vi "task 3.vi"() -> ()   [LabVIEW 2017]
uses:
  <vilib>/DAQmx/write.llb/DAQmx Write (Analog DBL 1Chan 1Samp).vi
  <vilib>/DAQmx/create/channels.llb/DAQmx Create Channel (AO-Voltage-Basic).vi
  <vilib>/DAQmx/create/channels.llb/DAQmx Create Channel (DI-Digital Input).vi
  <vilib>/DAQmx/read.llb/DAQmx Read (Digital Bool 1Line 1Point).vi
  <vilib>/DAQmx/read.llb/DAQmx Read (Counter DBL 1Chan 1Samp).vi
  <vilib>/DAQmx/create/channels.llb/DAQmx Create Channel (CI-Count Edges).vi
  <vilib>/Simulation/Implementation/XNodeFramework/SimXNode/SimX.xnode
  <vilib>/Simulation/Model Libraries/PID/SIM PID.vi
  <vilib>/Simulation/Model Libraries/PID/SIM PID (Parallel).vi
  <vilib>/Simulation/Implementation/Shared/SIMSCR Execution Mode.ctl
  <vilib>/Simulation/Scripting/Companion Diagram/SimConfigNode/_simSolvers.ctl
  <vilib>/Simulation/Scripting/Companion Diagram/SimConfigNode/SimParams.ctl
  <vilib>/Simulation/Scripting/Companion Diagram/SimConfigNode/SimDog.xnode
  <vilib>/Simulation/Model Libraries/PID/SIM PID (Academic).vi
  <vilib>/Simulation/Implementation/Shared/SIM Bundle Sim Info.vi
  <vilib>/Simulation/Implementation/Shared/SIM Unbundle Sim Info.vi
  <vilib>/Simulation/Implementation/Shared/NILVSim_FinalizeModel.vi
  <vilib>/Simulation/Implementation/Shared/NILVSim_GetModelError.vi
  <vilib>/Simulation/Implementation/Shared/NILVSim_Initialize.vi
  <vilib>/Simulation/Utility/Implementation/NILVSim Get Time and IsAcceptedStep.vi
  <vilib>/Simulation/Implementation/Shared/NILVSim_Manager.vi
  <vilib>/Simulation/Implementation/Shared/NI_SIM_Implementation.lvlib
  <vilib>/Simulation/Implementation/Shared/NILVSIM_BeginStep.vi
  <vilib>/Simulation/Param Hierarchy/Typedefs/SIMPH Param Control Actions.ctl
  <vilib>/Simulation/Implementation/Shared/NILVSim_ParamChanged.vi
  <vilib>/Utility/error.llb/Clear Errors.vi
  <vilib>/Simulation/Implementation/Shared/SIMSH Read Queue.vi
panel:
  in  "rectrangle":bool
  in  "Circle":bool
  in  "Right-Down":bool
  in  "Left-Up":bool
  in  "Left-Down":bool
  in  "Right-Up":bool
  in  "right":bool
  in  "left":bool
  in  "motor 2":dbl(slide)=1.5 scale=-10.0..10.0
  in  "down":bool
  in  "up":bool
  in  "Numeric 2":dbl
  in  "Numeric":dbl
  in  "DAQmx Physical Channel 8":tag="Dev9/ao0"
  out "no of pulses 2":dbl format="%.2f"
  in  "DAQmx Physical Channel 7":tag="Dev9/ao0"
  out "no of pulses":dbl format="%.2f"
  out "Right":bool
  out "Bottom":bool
  out "Left":bool
  out "Top":bool
  in  "DAQmx Physical Channel 6":tag
  in  "DAQmx Physical Channel 5":tag
  in  "DAQmx Physical Channel 4":tag
  in  "DAQmx Physical Channel 3":tag
  in  "Motor stop":bool
  in  "DAQmx Physical Channel 2":tag="Dev9/ao0"
  in  "max Voltage":dbl
  in  "Min Voltage":dbl
  in  "DAQmx Physical Channel":tag="Dev9/ao0"
  in  "motor 1":dbl(slide)=1.5 scale=-10.0..10.0
  in  "stop":bool
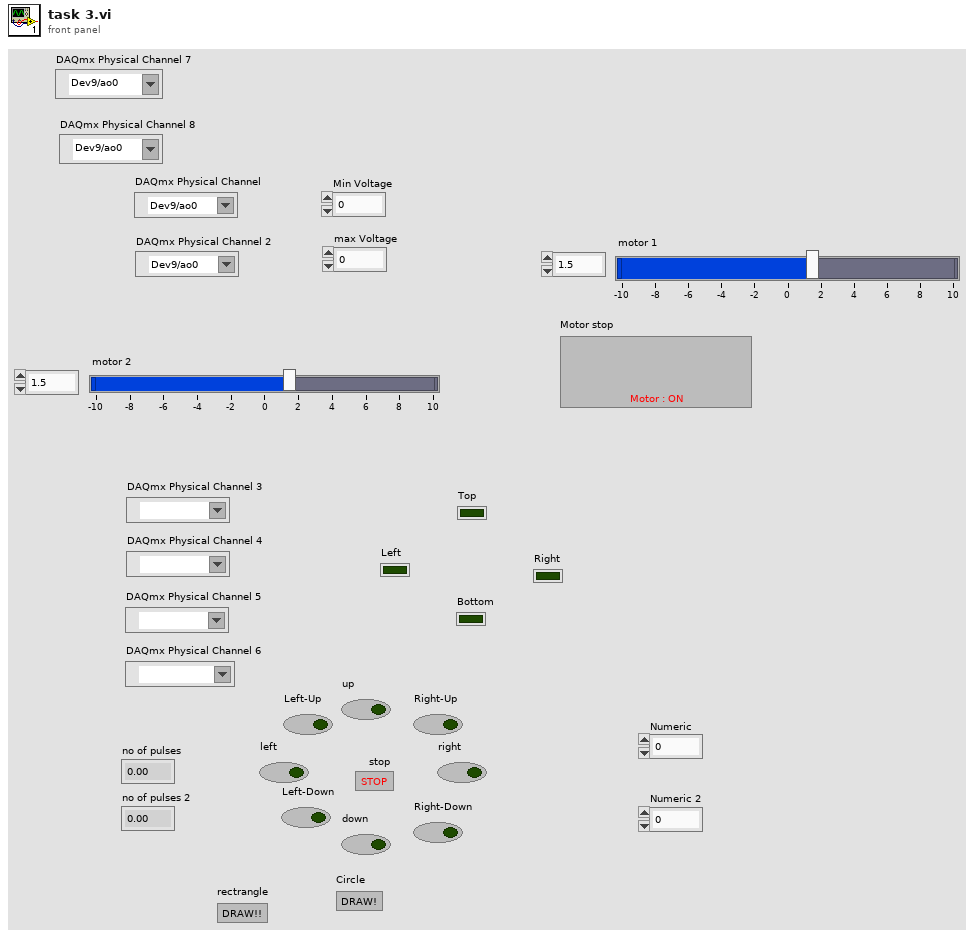
[diagram p1: front panel]
types:
  T1 = enum16{"Simulate to Completion", "Single Time-Step Simulation (Fixed Step Only)"}
  T2 = typedef "SIMSCR Execution Mode.ctl" = enum16{"Simulate to Completion", "Single Time-Step Simulation (Fixed Step Only)"}
  T3 = typedef "SIMPH Param Control Actions.ctl" = enum16{"get params", "set params"}
  T4 = cluster{"SIMSH Sim Time":dbl, "SIM PID Derivative Gain.vi":cluster{"output":dbl}, "SIM PID Derivative Gain.vi - SIMSH":cluster{"SIMSH Sim Time":dbl, "t 3":dbl, "Select 2":cluster{"s? t:f":dbl}, "Equal?":cluster{"x = y?":bool}, "Or":cluster{"x .or. y?":bool}, "Equal To 0?":cluster{"x = 0?":bool}}, "High Frequency [s] (Tf)":dbl, "Gain":cluster{"output":dbl}, "Summation":cluster{"Result":dbl}, "Integral Gain - series.vi":cluster{"output":dbl}, "Integral Gain - series.vi - SIMSH":cluster{"SIMSH Sim Time":dbl, "Select 2":cluster{"s? t:f":dbl}, "integral in gain?":bool, "Integrator":cluster{"output y(t)":dbl}, "Gain 2":cluster{"output":dbl}, "Select":cluster{"s? t:f":dbl}, "Equal To 0?":cluster{"x = 0?":bool}, "Reciprocal":cluster{"1/x":dbl}}}
  T5 = typedef "SimParams.ctl" = cluster{"Initial Time (s)":dbl, "Final Time (s)":dbl, "Step Size (s)":dbl, "ODE Solver":T6, "Minimum Step Size (s)":dbl, "Maximum Step Size (s)":dbl, "Relative Tolerance":dbl, "Absolute Tolerance":dbl, "Software Timing":bool, "Initial Step Size (s)":dbl, "Automatic Fixed Step Size?":bool, "Automatic Discrete Step Size?":bool, "Discrete Step Size (s)":dbl, "Calculate using Time Step":bool, "Solver Wired?":bool, "Prev.Frm.Expected End":u64, "Prev.Frm.Actual End":u64, "Prev.Frm.Finished Late?":bool, "Prev.Iter.Expected End":u64, "Prev.Iter.Actual End":u64, "Prev.Iter.Finished Late?":bool, "Expected Iteration Start":u64, "Actual Iteration Start":u64, "Expected Frame Start":u64, "Actual Frame Start":u64, "Source Name":string, "Name":string, "Period":i64, "Deadline":i64, "Offset":i64, "Start":i64, "Priority":i32, "Timeout":i32, "Processor":i32, "Mode":enum32{"No Change", "Process missed periods, maintain original phase", "Discard missed periods, maintain original phase", "Process missed periods, ignore original phase", "Discard missed periods, ignore original phase"}, "Wakeup reason":enum32{"Normal", "Aborted", "Asynchronous wakeup", "Timing source error", "Timed loop error", "Timeout"}, "Error":errorcluster, "Source Type":string, "Secondary Source Type":string, "Global End Time":u64, "Global Start Time":u64, "Full Solver Reset":bool, "Execution Mode":T2, "Nan/Inf Check":bool, "Custom Solver Library":string, "Solver Is Variable":bool, "custom solver name":string, "Signal Collection Decimation":u32}
  T6 = typedef "_simSolvers.ctl" = enum16{"Runge-Kutta 1 (Euler)", "Runge-Kutta 2", "Runge-Kutta 3", "Runge-Kutta 4", "Runge-Kutta 23 (variable)", "Runge-Kutta 45 (variable)", "BDF (variable)", "Adams-Moulton (variable)", "Rosenbrock (variable)", "Discrete States Only", "SDIRK 4 (variable)", "Radau 5 (variable)", "Radau 9 (variable)", "Radau 13 (variable)", "Radau [Variable Order] (variable)", "Gear's Method (variable)", "Linearizer", "State Query", "Trim Eval", "Custom Solver"}
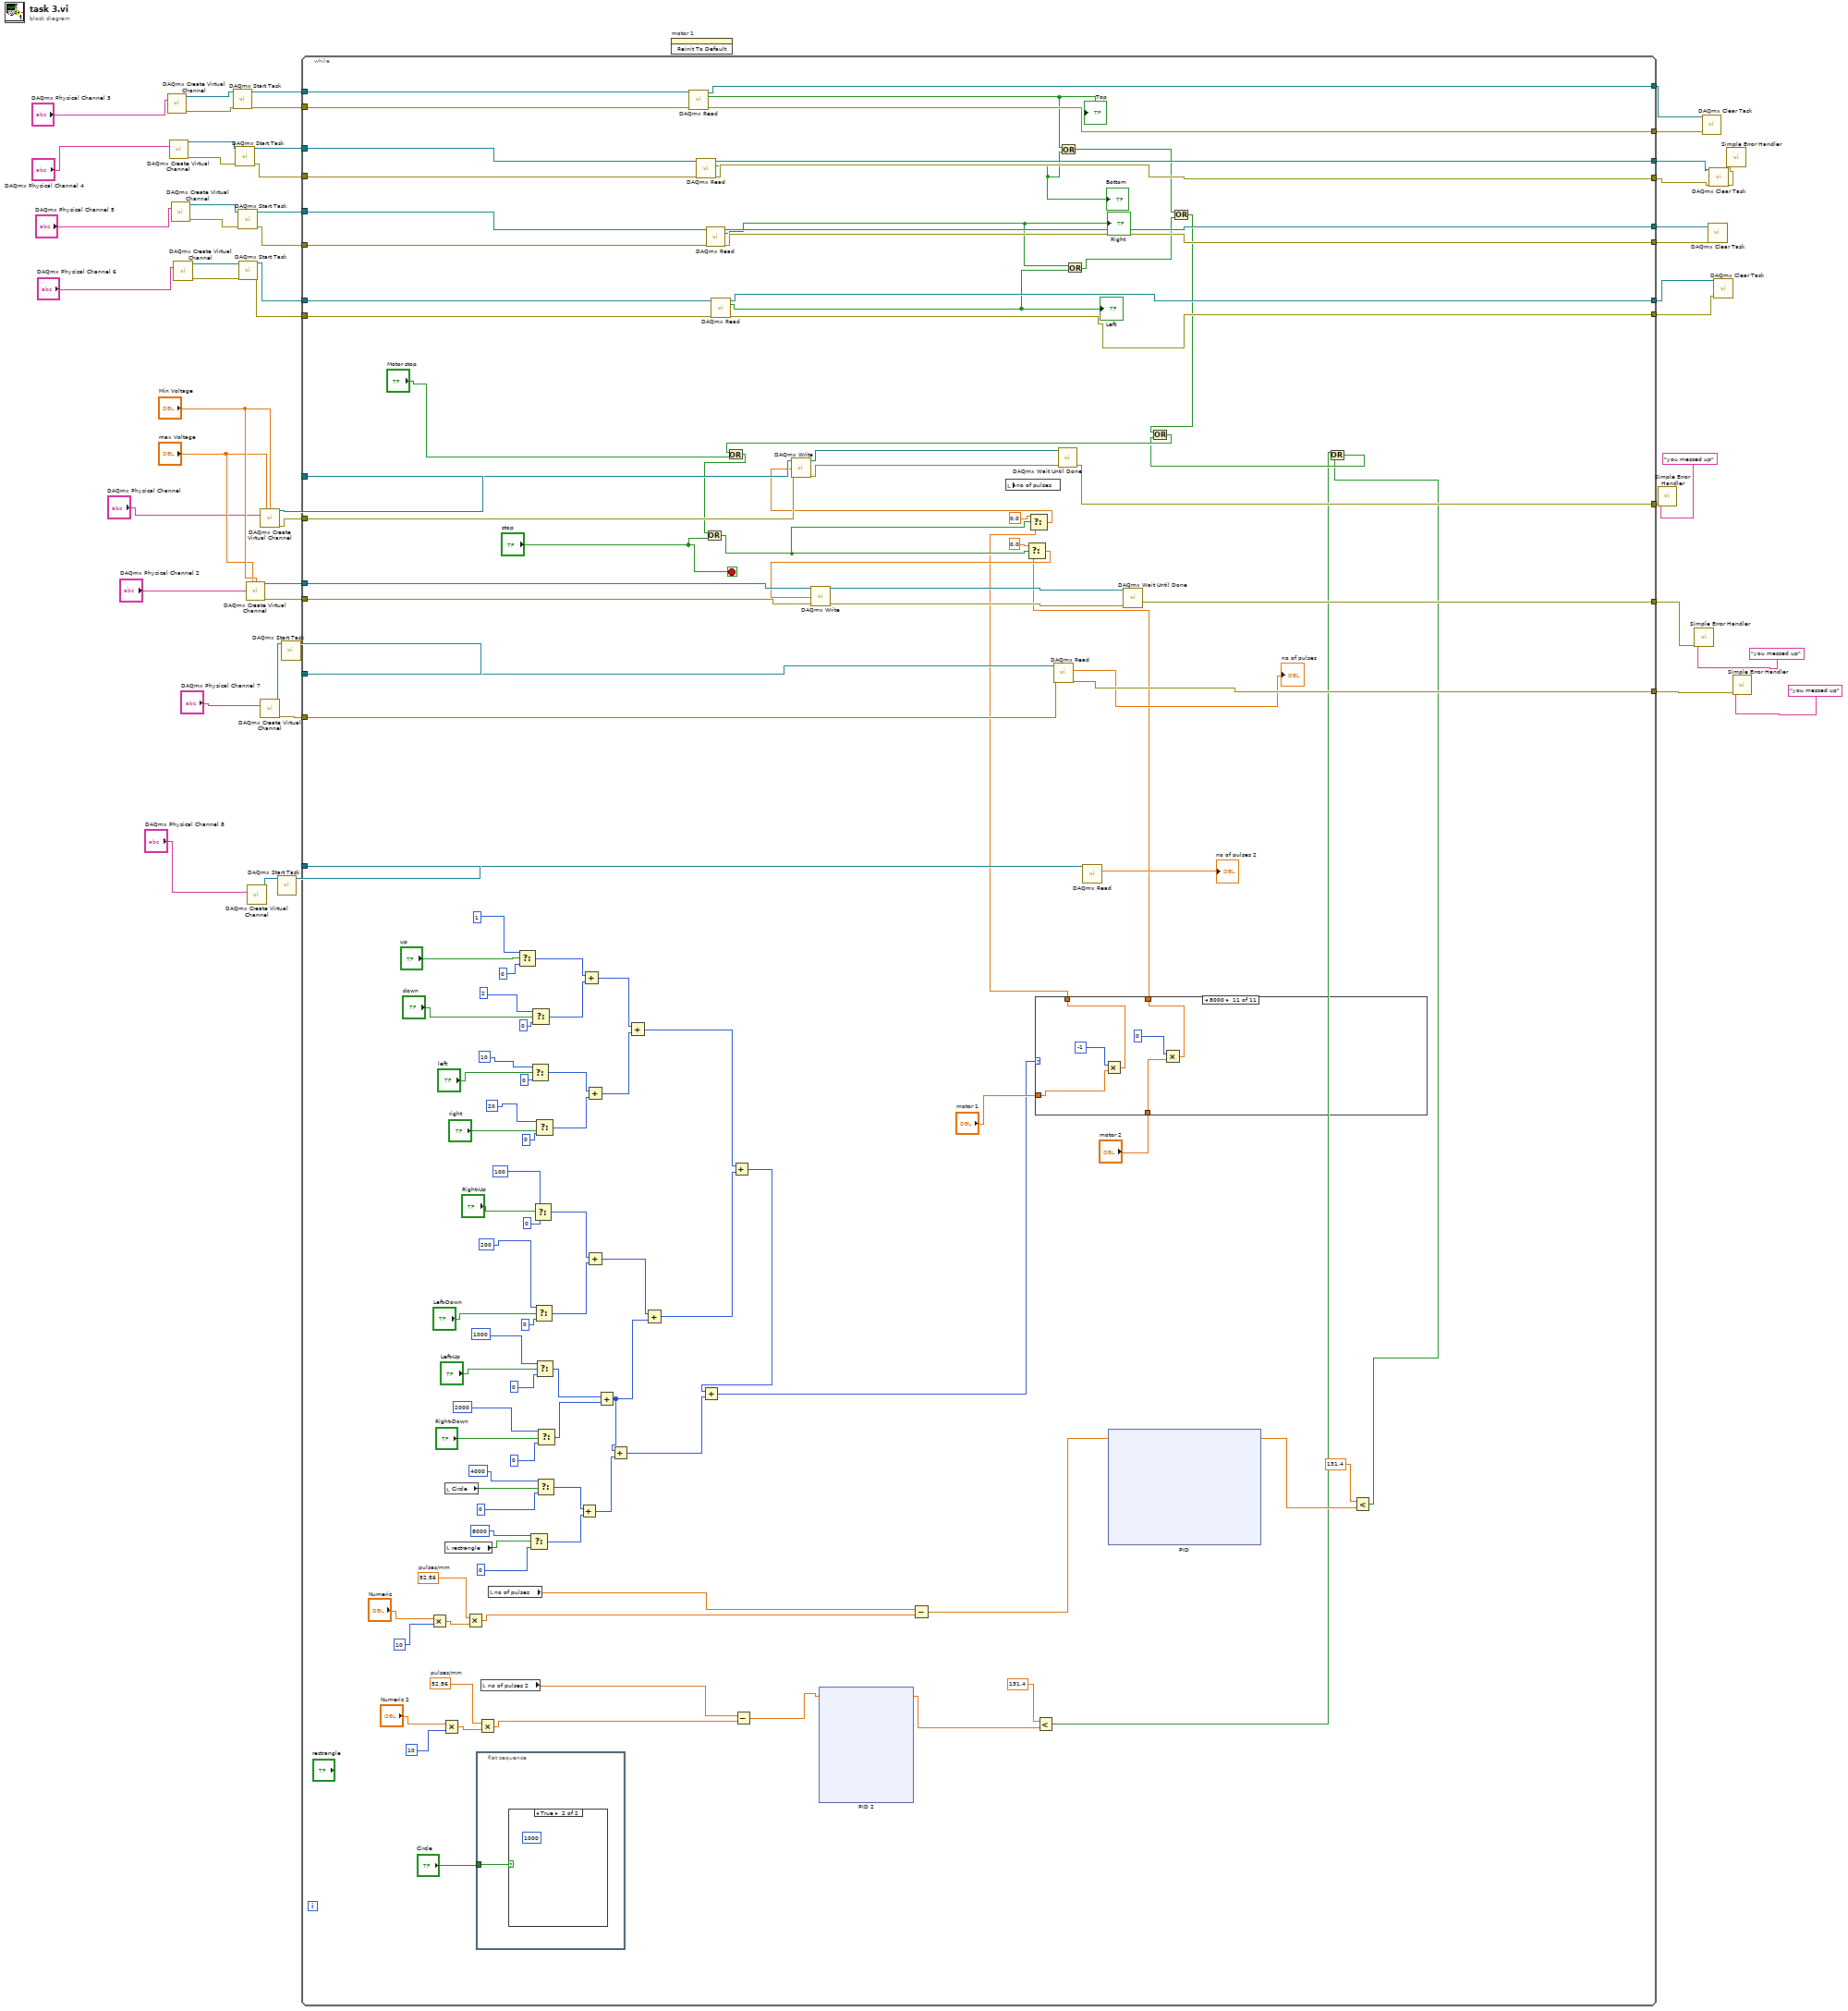
[diagram p0: block diagram]
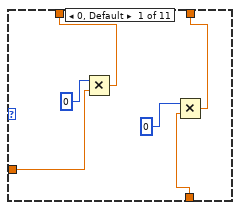
[diagram p3: hidden frame]
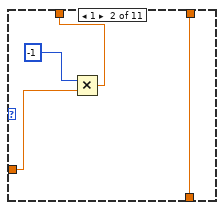
[diagram p4: hidden frame]
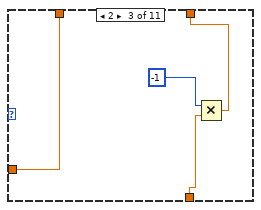
[diagram p5: hidden frame]
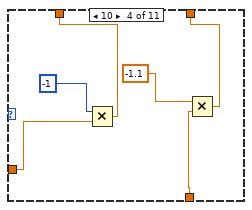
[diagram p6: hidden frame]
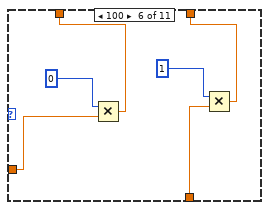
[diagram p8: hidden frame]
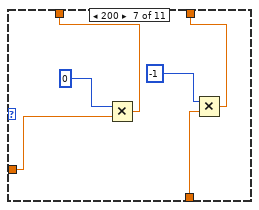
[diagram p9: hidden frame]
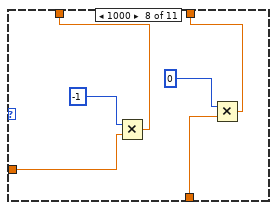
[diagram p10: hidden frame]
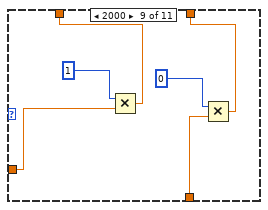
[diagram p11: hidden frame]
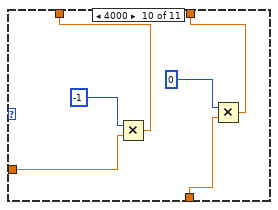
[diagram p12: hidden frame]
diagram:
  n1 = call-poly <vilib>:"DAQmx Create Virtual Channel.vi"("lines"="DAQmx Physical Channel 3") -> ("task out"=w36:refnum<k21>, "error out"=w32:errorcluster)  [unwired: 13 in]
  n2 = call-poly <vilib>:"DAQmx Create Virtual Channel.vi"("lines"="DAQmx Physical Channel 4") -> ("task out"=w35:refnum<k21>, "error out"=w31:errorcluster)  [unwired: 13 in]
  n3 = call-poly <vilib>:"DAQmx Create Virtual Channel.vi"("lines"="DAQmx Physical Channel 5") -> ("task out"=w34:refnum<k21>, "error out"=w30:errorcluster)  [unwired: 13 in]
  n4 = call-poly <vilib>:"DAQmx Create Virtual Channel.vi"("lines"="DAQmx Physical Channel 6") -> ("task out"=w33:refnum<k21>, "error out"=w29:errorcluster)  [unwired: 13 in]
  n5 = call <vilib>:"DAQmx Start Task.vi"("task/channels in"=w36, "error in"=w32) -> ("task out"=w28:refnum<k21>, "error out"=w26:errorcluster)  [unwired: 12 in]
  n6 = call <vilib>:"DAQmx Start Task.vi"("task/channels in"=w35, "error in"=w31) -> ("task out"=w24:refnum<k21>, "error out"=w21:errorcluster)  [unwired: 12 in]
  n7 = call <vilib>:"DAQmx Start Task.vi"("task/channels in"=w34, "error in"=w30) -> ("task out"=w23:refnum<k21>, "error out"=w20:errorcluster)  [unwired: 12 in]
  n8 = call <vilib>:"DAQmx Start Task.vi"("task/channels in"=w33, "error in"=w29) -> ("task out"=w22:refnum<k21>, "error out"=w19:errorcluster)  [unwired: 12 in]
  n9 = call-poly <vilib>:"DAQmx Create Virtual Channel.vi"("maximum value"="max Voltage", "minimum value"="Min Voltage", "physical channels"="DAQmx Physical Channel 2") -> ("task out"=w46:refnum<k21>, "error out"=w42:errorcluster)  [unwired: 11 in]
  n10 = call-poly <vilib>:"DAQmx Create Virtual Channel.vi"("counter"="DAQmx Physical Channel 8") -> ("task out"=w4:refnum<k21>)  [unwired: 13 in, 1 out]
  n11 = call-poly <vilib>:"DAQmx Create Virtual Channel.vi"("maximum value"="max Voltage", "minimum value"="Min Voltage", "physical channels"="DAQmx Physical Channel") -> ("task out"=w49:refnum<k21>, "error out"=w41:errorcluster)  [unwired: 11 in]
  n12 = call-poly <vilib>:"DAQmx Create Virtual Channel.vi"("counter"="DAQmx Physical Channel 7") -> ("task out"=w6:refnum<k21>, "error out"=w7:errorcluster)  [unwired: 13 in]
  n13 = call <vilib>:"DAQmx Start Task.vi"("task/channels in"=w4) -> ("task out"=w3:refnum<k21>)  [unwired: 13 in, 1 out]
  n14 = call <vilib>:"DAQmx Start Task.vi"("task/channels in"=w6) -> ("task out"=w5:refnum<k21>)  [unwired: 13 in, 1 out]
  n15 = while {
    tunnel: w49 -> [w174]
    tunnel: [w171] -> w48
    tunnel: w46 -> [w168]
    tunnel: [w167] -> w45
    tunnel: w42 -> [w165]
    tunnel: w41 -> [w164]
    tunnel: w28 -> [w158]
    tunnel: [w157] -> w27
    tunnel: w26 -> [w156]
    tunnel: [w155] -> w25
    tunnel: w24 -> [w154]
    tunnel: w23 -> [w153]
    tunnel: w22 -> [w152]
    tunnel: w21 -> [w151]
    tunnel: w20 -> [w150]
    tunnel: w19 -> [w149]
    tunnel: [w148] -> w18
    tunnel: [w147] -> w17
    tunnel: [w146] -> w16
    tunnel: [w145] -> w15
    tunnel: [w144] -> w14
    tunnel: [w143] -> w13
    tunnel: [w142] -> w10
    tunnel: w5 -> [w141]
    tunnel: w7 -> [w140]
    tunnel: w3 -> [w131]
    stop <- "stop" stop-if-true
    w121 = 52.56  # pulses/mm
    w126 = 52.56  # pulses/mm
    n16 = Multiply(x="Numeric", y=10) -> (x*y=w125:dbl)
    n17 = Multiply(x="Numeric 2", y=10) -> (x*y=w124:dbl)
    n18 = local read "Circle"() -> (w63:bool)
    n19 = local read "rectrangle"() -> (w61:bool)
    n20 = Multiply(x=w126, y=w125) -> (x*y=w114:dbl)
    n21 = flat-sequence {
      tunnel: "Circle" -> [w175]
      frame #0 {
        n22 = case shown="True" w175 {
          frame False {
          }
          frame True {
            (unwired) 1000
          }
        }
      }
    }
    n23 = Multiply(x=w121, y=w124) -> (x*y=w108:dbl)
    n24 = local read "no of pulses 2"() -> (w109:dbl)
    n25 = local read "no of pulses"() -> (w115:dbl)
    n26 = Select(t=1, s="up", f=0) -> (s? t:f=w88:i32)
    n27 = Select(t=8000, s=w61, f=0) -> (s? t:f=w58:i32)
    n28 = Select(t=10, s="left", f=0) -> (s? t:f=w86:i32)
    n29 = Select(t=2, s="down", f=0) -> (s? t:f=w87:i32)
    n30 = Select(t=100, s="Right-Up", f=0) -> (s? t:f=w84:i32)
    n31 = Select(t=200, s="Left-Down", f=0) -> (s? t:f=w83:i32)
    n32 = Select(t=20, s="right", f=0) -> (s? t:f=w85:i32)
    n33 = Select(t=1000, s="Left-Up", f=0) -> (s? t:f=w82:i32)
    n34 = Select(t=4000, s=w63, f=0) -> (s? t:f=w59:i32)
    n35 = Select(t=2000, s="Right-Down", f=0) -> (s? t:f=w66:i32)
    n36 = Add(x=w59, y=w58) -> (x+y=w56:i32)
    n37 = Add(x=w88, y=w87) -> (x+y=w81:i32)
    n38 = Add(x=w86, y=w85) -> (x+y=w80:i32)
    n39 = Add(x=w84, y=w83) -> (x+y=w79:i32)
    n40 = Add(x=w82, y=w66) -> (x+y=w57:i32)
    n41 = Add(x=w57, y=w56) -> (x+y=w55:i32)
    n42 = Add(x=w81, y=w80) -> (x+y=w78:i32)
    n43 = Add(x=w79, y=w57) -> (x+y=w54:i32)
    n44 = call-poly <vilib>:"DAQmx Read.vi"("task/channels in"=w158, "error in"=w156) -> ("task out"=w157:refnum<k21>, "data"=w139:bool, "error out"=w155:errorcluster)  [unwired: 11 in]
    "Top" <- w139
    n45 = call-poly <vilib>:"DAQmx Read.vi"("task/channels in"=w154, "error in"=w151) -> ("task out"=w148:refnum<k21>, "data"=w138:bool, "error out"=w145:errorcluster)  [unwired: 11 in]
    "Bottom" <- w138
    n46 = call-poly <vilib>:"DAQmx Read.vi"("task/channels in"=w153, "error in"=w150) -> ("task out"=w147:refnum<k21>, "data"=w136:bool, "error out"=w144:errorcluster)  [unwired: 11 in]
    "Right" <- w136
    n47 = call-poly <vilib>:"DAQmx Read.vi"("task/channels in"=w152, "error in"=w149) -> ("task out"=w146:refnum<k21>, "data"=w135:bool, "error out"=w143:errorcluster)  [unwired: 11 in]
    "Left" <- w135
    n48 = Add(x=w78, y=w54) -> (x+y=w53:i32)
    n49 = Add(x=w53, y=w55) -> (x+y=w52:i32)
    n50 = Subtract(x=w109, y=w108) -> (x-y=w107:dbl)
    n51 = xnode "PID 2"("Error"=w107) -> ("Output"=w105:dbl)  [unwired: 2 in, 11 out]
    n52 = Subtract(x=w115, y=w114) -> (x-y=w113:dbl)
    n53 = local read "no of pulses"() -> ()  [unwired: 1 in]
    n54 = case shown="8000" w52 {
      tunnel: "motor 1" -> [w674 w677 w680 w687 w691 w695 w701 w707 w713 w718 w725]
      tunnel: "motor 2" -> [w671 w679 w682 w685 w690 w693 w699 w705 w711 w719 w724]
      tunnel: [w670 w679 w681 w684 w690 w692 w698 w704 w710 w716 w723] -> w69
      tunnel: [w673 w676 w680 w686 w691 w694 w700 w706 w712 w717 w722] -> w68
      frame 0, Default {
        n55 = Multiply(x=0, y=w674) -> (x*y=w673:dbl)
        n56 = Multiply(x=0, y=w671) -> (x*y=w670:dbl)
      }
      frame 1 {
        n57 = Multiply(x=-1, y=w677) -> (x*y=w676:dbl)
      }
      frame 2 {
        n58 = Multiply(x=-1, y=w682) -> (x*y=w681:dbl)
      }
      frame 10 {
        n59 = Multiply(x=-1, y=w687) -> (x*y=w686:dbl)
        n60 = Multiply(x=-1.1, y=w685) -> (x*y=w684:dbl)
      }
      frame 20 {
      }
      frame 100 {
        n61 = Multiply(x=0, y=w695) -> (x*y=w694:dbl)
        n62 = Multiply(x=1, y=w693) -> (x*y=w692:dbl)
      }
      frame 200 {
        n63 = Multiply(x=0, y=w701) -> (x*y=w700:dbl)
        n64 = Multiply(x=-1, y=w699) -> (x*y=w698:dbl)
      }
      frame 1000 {
        n65 = Multiply(x=-1, y=w707) -> (x*y=w706:dbl)
        n66 = Multiply(x=0, y=w705) -> (x*y=w704:dbl)
      }
      frame 2000 {
        n67 = Multiply(x=1, y=w713) -> (x*y=w712:dbl)
        n68 = Multiply(x=0, y=w711) -> (x*y=w710:dbl)
      }
      frame 4000 {
        n69 = Multiply(x=-1, y=w718) -> (x*y=w717:dbl)
        n70 = Multiply(x=0, y=w719) -> (x*y=w716:dbl)
      }
      frame 8000 {
        n71 = Multiply(x=-1, y=w725) -> (x*y=w722:dbl)
        n72 = Multiply(x=0, y=w724) -> (x*y=w723:dbl)
      }
    }
    n73 = Less?(x=131.4, y=w105) -> (x < y?=w104:bool)
    n74 = call-poly <vilib>:"DAQmx Read.vi"("task/channels in"=w141, "error in"=w140) -> ("data"=→"no of pulses":dbl, "error out"=w142:errorcluster)  [unwired: 11 in, 1 out]
    n75 = Or(x=w139, y=w138) -> (x .or. y?=w137:bool)
    n76 = Or(x=w136, y=w135) -> (x .or. y?=w134:bool)
    n77 = call-poly <vilib>:"DAQmx Read.vi"("task/channels in"=w131) -> ("data"=→"no of pulses 2":dbl)  [unwired: 12 in, 2 out]
    n78 = xnode "PID"("Error"=w113) -> ("Output"=w112:dbl)  [unwired: 2 in, 11 out]
    n79 = Or(x=w137, y=w134) -> (x .or. y?=w130:bool)
    n80 = Less?(x=131.4, y=w112) -> (x < y?=w110:bool)
    n81 = Or(x=w104, y=w110) -> (x .or. y?=w120:bool)
    n82 = Or(x=w130, y=w120) -> (x .or. y?=w129:bool)
    n83 = Or(x=w129, y="Motor stop") -> (x .or. y?=w133:bool)
    n84 = Or(x=w133, y="stop") -> (x .or. y?=w162:bool)
    n85 = Select(t=0.0, s=w162, f=w69) -> (s? t:f=w159:dbl)
    n86 = call-poly <vilib>:"DAQmx Write.vi"("task/channels in"=w168, "data"=w159, "error in"=w165) -> ("task out"=w169:refnum<k21>, "error out"=w170:errorcluster)  [unwired: 10 in, 1 out]
    n87 = Select(t=0.0 ("s? t:f"), s=w162, f=w68) -> (s? t:f=w160:dbl)
    n88 = call-poly <vilib>:"DAQmx Write.vi"("task/channels in"=w174, "data"=w160, "error in"=w164) -> ("task out"=w173:refnum<k21>, "error out"=w172:errorcluster)  [unwired: 10 in, 1 out]
    n89 = call <vilib>:"DAQmx Wait Until Done.vi"("task/channels in"=w173, "error in"=w172) -> ("error out"=w171:errorcluster)  [unwired: 12 in, 1 out]
    n90 = call <vilib>:"DAQmx Wait Until Done.vi"("task/channels in"=w169, "error in"=w170) -> ("error out"=w167:errorcluster)  [unwired: 12 in, 1 out]
  }
  n91 = invoke on="motor 1" class="Slide (strict)" method="Reinit To Default"() -> ()  [unwired: 3 in, 3 out]
  n92 = call <vilib>:"Simple Error Handler.vi"("error source (\" \")"="you messed up" ("error source (\" \")"), "error in (no error)"=w48) -> ()  [unwired: 3 in, 5 out]
  n93 = call <vilib>:"Simple Error Handler.vi"("error source (\" \")"="you messed up" ("error source (\" \")"), "error in (no error)"=w45) -> ()  [unwired: 3 in, 5 out]
  n94 = call <vilib>:"DAQmx Clear Task.vi"("task in"=w27, "error in"=w25) -> ()  [unwired: 13 in, 1 out]
  n95 = call <vilib>:"DAQmx Clear Task.vi"("task in"=w17, "error in"=w14) -> ()  [unwired: 13 in, 1 out]
  n96 = call <vilib>:"DAQmx Clear Task.vi"("task in"=w18, "error in"=w15) -> ("error out"=w12:errorcluster)  [unwired: 13 in]
  n97 = call <vilib>:"DAQmx Clear Task.vi"("task in"=w16, "error in"=w13) -> ()  [unwired: 13 in, 1 out]
  n98 = call <vilib>:"Simple Error Handler.vi"("error in (no error)"=w12) -> ()  [unwired: 4 in, 5 out]
  n99 = call <vilib>:"Simple Error Handler.vi"("error source (\" \")"="you messed up" ("error source (\" \")"), "error in (no error)"=w10) -> ()  [unwired: 3 in, 5 out]
